vi "newsubvi Robot Jog Control.vi"(1 "VISA In":refnum<visa-resource-name>="COM4") -> (0 "VISA Out":refnum<visa-resource-name>="COM4")   [LabVIEW 2012]
panel:
  in  "RobotJogSpeed":enum32{"Slow", "Fast"}(radio)
  in  "RobotDn":bool
  in  "RobotUp":bool
  in  "RobotNear":bool
  in  "RobotFar":bool
  in  "RobotRight":bool
  in  "RobotLeft":bool
  in  "stop":bool
  # "Jog Speed"
  # "Jog Control"
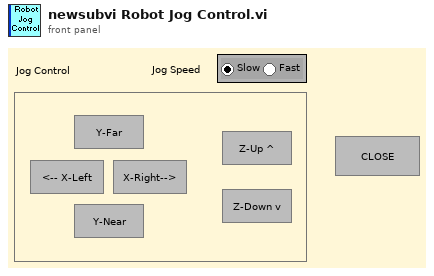
[diagram p1: front panel]
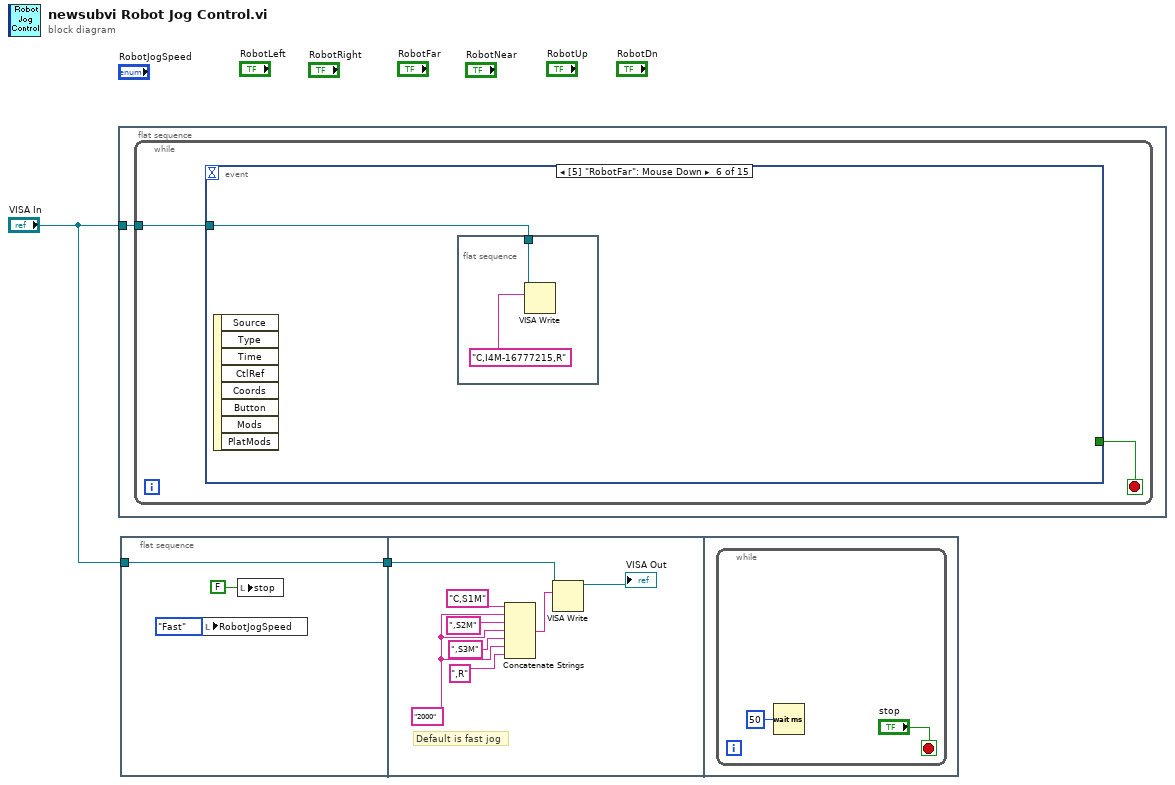
[diagram p0: block diagram]
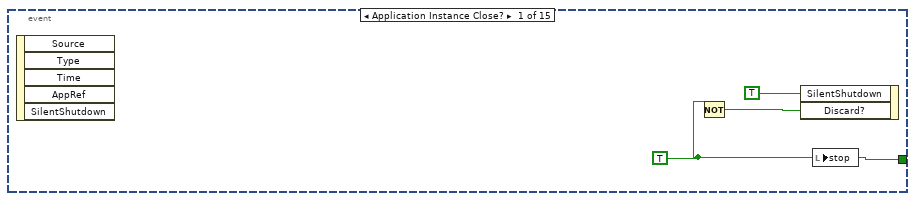
[diagram p2: hidden frame]
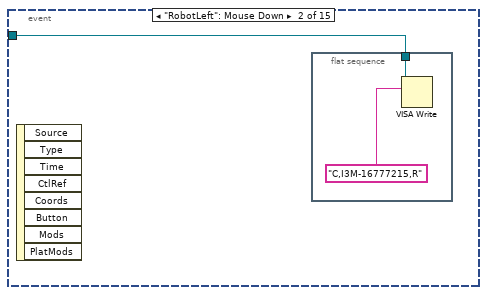
[diagram p3: hidden frame]
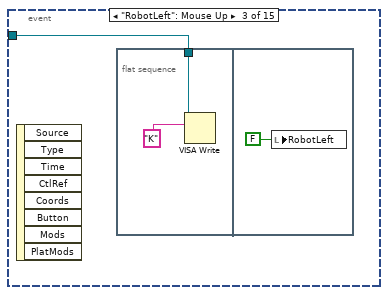
[diagram p4: hidden frame]
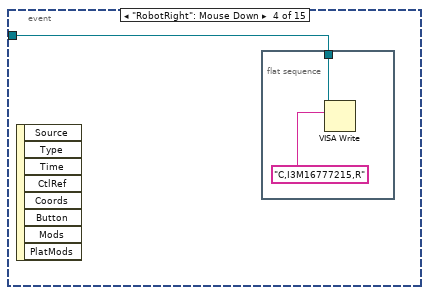
[diagram p5: hidden frame]
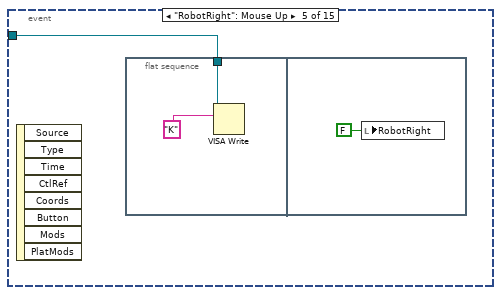
[diagram p6: hidden frame]
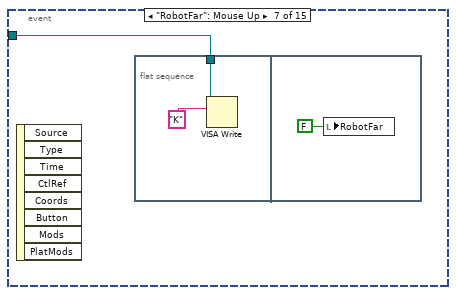
[diagram p7: hidden frame]
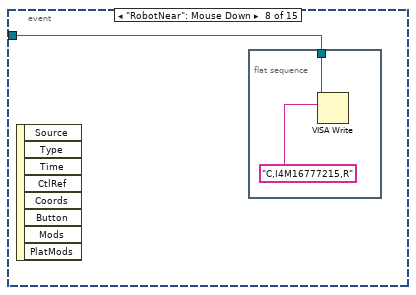
[diagram p8: hidden frame]
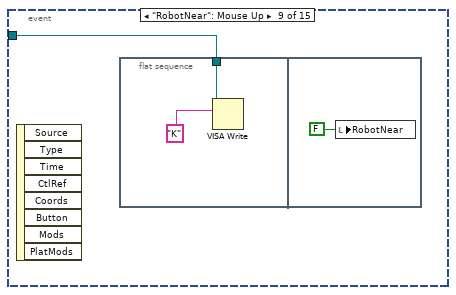
[diagram p9: hidden frame]
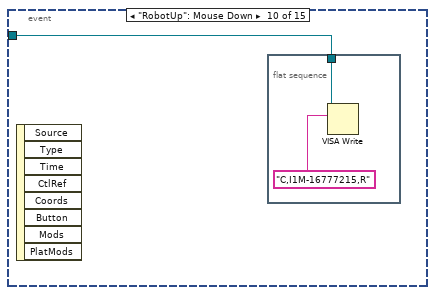
[diagram p10: hidden frame]
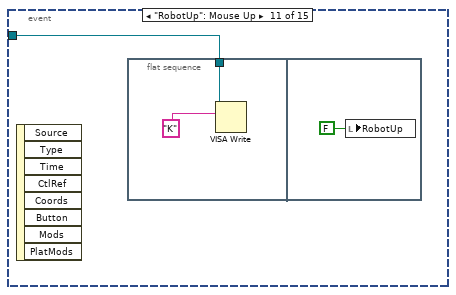
[diagram p11: hidden frame]
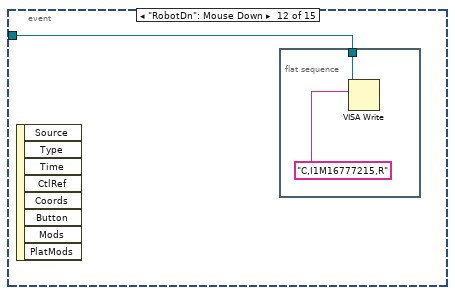
[diagram p12: hidden frame]
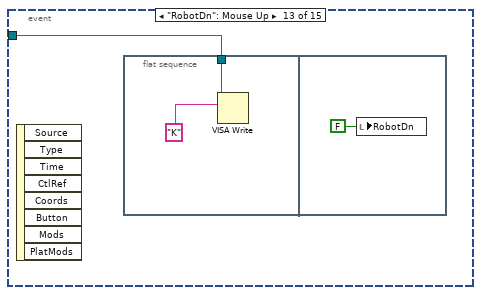
[diagram p13: hidden frame]
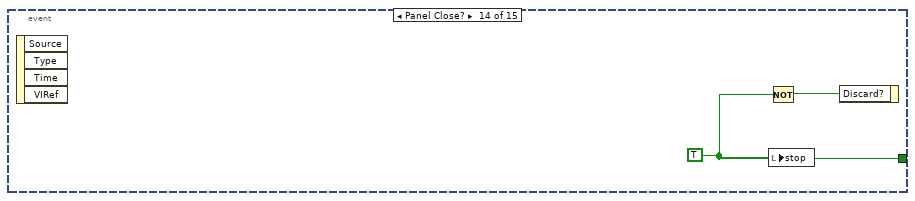
[diagram p14: hidden frame]
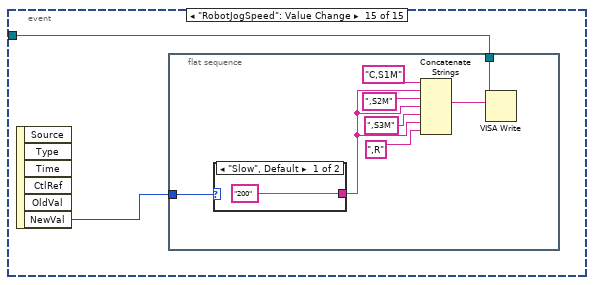
[diagram p15: hidden frame]
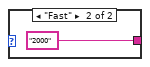
[diagram p16: hidden frame]
diagram:
  n1 = flat-sequence {
    tunnel: "VISA In" -> [w3]
    frame #0 {
      n2 = while {
        tunnel: w3 -> [w4]
        stop <- w5 stop-if-true
        n3 = event shown="[5] \"RobotFar\": Mouse Down" {
          selector: _ -> [_ _ _ _ _ _ _ _ _ _ _ _ _ _ _]
          dyn-events: _ -> [_ _ _ _ _ _ _ _ _ _ _ _ _ _ _]
          timeout: _ -> [_ _ _ _ _ _ _ _ _ _ _ _ _ _ _]
          tunnel: [w6 _ _ _ _ _ _ _ _ _ _ _ _ w51 _] -> w5
          tunnel: w4 -> [_ w9 w12 w16 w19 w23 w26 w30 w33 w37 w40 w44 w47 _ w53]
          event Application Instance Close? {
            w6 = TRUE
            n4 = event-data() -> ()  [unwired: 6 out]
            n5 = Not(x=w6) -> (.not. x?=w8:bool)
            n6 = event-data("SilentShutdown"=TRUE, "Discard?"=w8) -> ()  [unwired: 1 in, 1 out]
            n7 = local write "stop"(w6) -> ()
          }
          event "RobotLeft": Mouse Down {
            n8 = event-data() -> ()  [unwired: 9 out]
            n9 = flat-sequence {
              tunnel: w9 -> [w11]
              frame #0 {
                n10 = VISA Write(VISA resource name=w11, write buffer="C,I3M-16777215,R" ("Text to Send")) -> ()  [unwired: 1 in, 3 out]
              }
            }
          }
          event "RobotLeft": Mouse Up {
            n11 = event-data() -> ()  [unwired: 9 out]
            n12 = flat-sequence {
              tunnel: w12 -> [w14]
              frame #0 {
                n13 = VISA Write(VISA resource name=w14, write buffer="K" ("Text to Send")) -> ()  [unwired: 1 in, 3 out]
              }
              frame #1 {
                n14 = local write "RobotLeft"(FALSE ("RobotLeft")) -> ()
              }
            }
          }
          event "RobotRight": Mouse Down {
            n15 = event-data() -> ()  [unwired: 9 out]
            n16 = flat-sequence {
              tunnel: w16 -> [w18]
              frame #0 {
                n17 = VISA Write(VISA resource name=w18, write buffer="C,I3M16777215,R" ("Text to Send")) -> ()  [unwired: 1 in, 3 out]
              }
            }
          }
          event "RobotRight": Mouse Up {
            n18 = event-data() -> ()  [unwired: 9 out]
            n19 = flat-sequence {
              tunnel: w19 -> [w21]
              frame #0 {
                n20 = VISA Write(VISA resource name=w21, write buffer="K" ("Text to Send")) -> ()  [unwired: 1 in, 3 out]
              }
              frame #1 {
                n21 = local write "RobotRight"(FALSE ("RobotRight")) -> ()
              }
            }
          }
          event "RobotFar": Mouse Down {
            n22 = event-data() -> ()  [unwired: 9 out]
            n23 = flat-sequence {
              tunnel: w23 -> [w25]
              frame #0 {
                n24 = VISA Write(VISA resource name=w25, write buffer="C,I4M-16777215,R" ("Text to Send")) -> ()  [unwired: 1 in, 3 out]
              }
            }
          }
          event "RobotFar": Mouse Up {
            n25 = event-data() -> ()  [unwired: 9 out]
            n26 = flat-sequence {
              tunnel: w26 -> [w28]
              frame #0 {
                n27 = VISA Write(VISA resource name=w28, write buffer="K" ("Text to Send")) -> ()  [unwired: 1 in, 3 out]
              }
              frame #1 {
                n28 = local write "RobotFar"(FALSE ("RobotFar")) -> ()
              }
            }
          }
          event "RobotNear": Mouse Down {
            n29 = event-data() -> ()  [unwired: 9 out]
            n30 = flat-sequence {
              tunnel: w30 -> [w32]
              frame #0 {
                n31 = VISA Write(VISA resource name=w32, write buffer="C,I4M16777215,R" ("Text to Send")) -> ()  [unwired: 1 in, 3 out]
              }
            }
          }
          event "RobotNear": Mouse Up {
            n32 = event-data() -> ()  [unwired: 9 out]
            n33 = flat-sequence {
              tunnel: w33 -> [w35]
              frame #0 {
                n34 = VISA Write(VISA resource name=w35, write buffer="K" ("Text to Send")) -> ()  [unwired: 1 in, 3 out]
              }
              frame #1 {
                n35 = local write "RobotNear"(FALSE ("RobotNear")) -> ()
              }
            }
          }
          event "RobotUp": Mouse Down {
            n36 = event-data() -> ()  [unwired: 9 out]
            n37 = flat-sequence {
              tunnel: w37 -> [w39]
              frame #0 {
                n38 = VISA Write(VISA resource name=w39, write buffer="C,I1M-16777215,R" ("Text to Send")) -> ()  [unwired: 1 in, 3 out]
              }
            }
          }
          event "RobotUp": Mouse Up {
            n39 = event-data() -> ()  [unwired: 9 out]
            n40 = flat-sequence {
              tunnel: w40 -> [w42]
              frame #0 {
                n41 = VISA Write(VISA resource name=w42, write buffer="K" ("Text to Send")) -> ()  [unwired: 1 in, 3 out]
              }
              frame #1 {
                n42 = local write "RobotUp"(FALSE ("RobotUp")) -> ()
              }
            }
          }
          event "RobotDn": Mouse Down {
            n43 = event-data() -> ()  [unwired: 9 out]
            n44 = flat-sequence {
              tunnel: w44 -> [w46]
              frame #0 {
                n45 = VISA Write(VISA resource name=w46, write buffer="C,I1M16777215,R" ("Text to Send")) -> ()  [unwired: 1 in, 3 out]
              }
            }
          }
          event "RobotDn": Mouse Up {
            n46 = event-data() -> ()  [unwired: 9 out]
            n47 = flat-sequence {
              tunnel: w47 -> [w49]
              frame #0 {
                n48 = VISA Write(VISA resource name=w49, write buffer="K" ("Text to Send")) -> ()  [unwired: 1 in, 3 out]
              }
              frame #1 {
                n49 = local write "RobotDn"(FALSE ("RobotDn")) -> ()
              }
            }
          }
          event Panel Close? {
            w51 = TRUE
            n50 = event-data() -> ()  [unwired: 5 out]
            n51 = Not(x=w51) -> (.not. x?=w52:bool)
            n52 = local write "stop"(w51) -> ()
            n53 = event-data("Discard?"=w52) -> ()  [unwired: 1 in, 1 out]
          }
          event "RobotJogSpeed": Value Change {
            n54 = event-data() -> ("NewVal"=w54:enum32{"Slow", "Fast"})  [unwired: 6 out]
            n55 = flat-sequence {
              tunnel: w54 -> [w61]
              tunnel: w53 -> [w56]
              frame #0 {
                n56 = case shown="\"Slow\", Default" w61 {
                  tunnel: ["200" "2000"] -> w58
                  frame "Slow", Default {
                  }
                  frame "Fast" {
                  }
                }
                n57 = Concatenate Strings("C,S1M" ("string"), w58, ",S2M" ("string"), w58, ",S3M" ("string"), w58, ",R" ("string")) -> (w55:string)
                n58 = VISA Write(VISA resource name=w56, write buffer=w55) -> ()  [unwired: 1 in, 3 out]
              }
            }
          }
        }
      }
    }
  }
  n59 = flat-sequence {
    tunnel: [w65] -> w2
    tunnel: "VISA In" -> [w65]
    tunnel: w2 -> [w69]
    frame #0 {
      n60 = local write "RobotJogSpeed"(enum32{"Slow", "Fast"}."Fast" ("RobotJogSpeed")) -> ()
      n61 = local write "stop"(FALSE ("stop")) -> ()
    }
    frame #1 {
      w71 = "2000"
      # "Default is fast jog"
      n62 = Concatenate Strings("C,S1M" ("string"), w71, ",S2M" ("string"), w71, ",S3M" ("string"), w71, ",R" ("string")) -> (w70:string)
      n63 = VISA Write(VISA resource name=w69, write buffer=w70) -> (VISA resource name out=→"VISA Out":refnum<visa-resource-name>)  [unwired: 1 in, 2 out]
    }
    frame #2 {
      n64 = while {
        stop <- "stop" stop-if-true
        n65 = Wait (ms)(milliseconds to wait=u32 50) -> ()  [unwired: 1 out]
      }
    }
  }
